vi "imaging gate sweep.vi"() -> ()   [LabVIEW 2021]
uses:
  <userlib>/Nanonis Prog Interface V5/Nanonis Prog Interface.lvlib
panel:
  in  "Home\nafter?":bool
  in  "?":bool
  in  "milliseconds to wait":u32
  in  "Direction: \nUp\n\n\nDown":bool=TRUE
  in  "Serie name":string caption="Basename (empty= no change)"
  in  "Gate increment (V)":dbl
  in  "End gate (V)":dbl
  in  "Start gate (V)":dbl
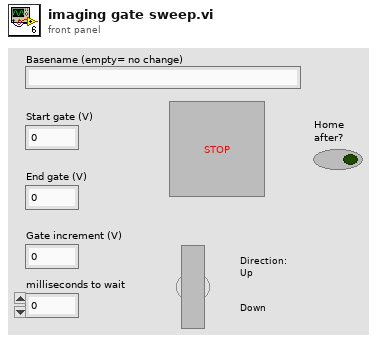
[diagram p1: front panel]
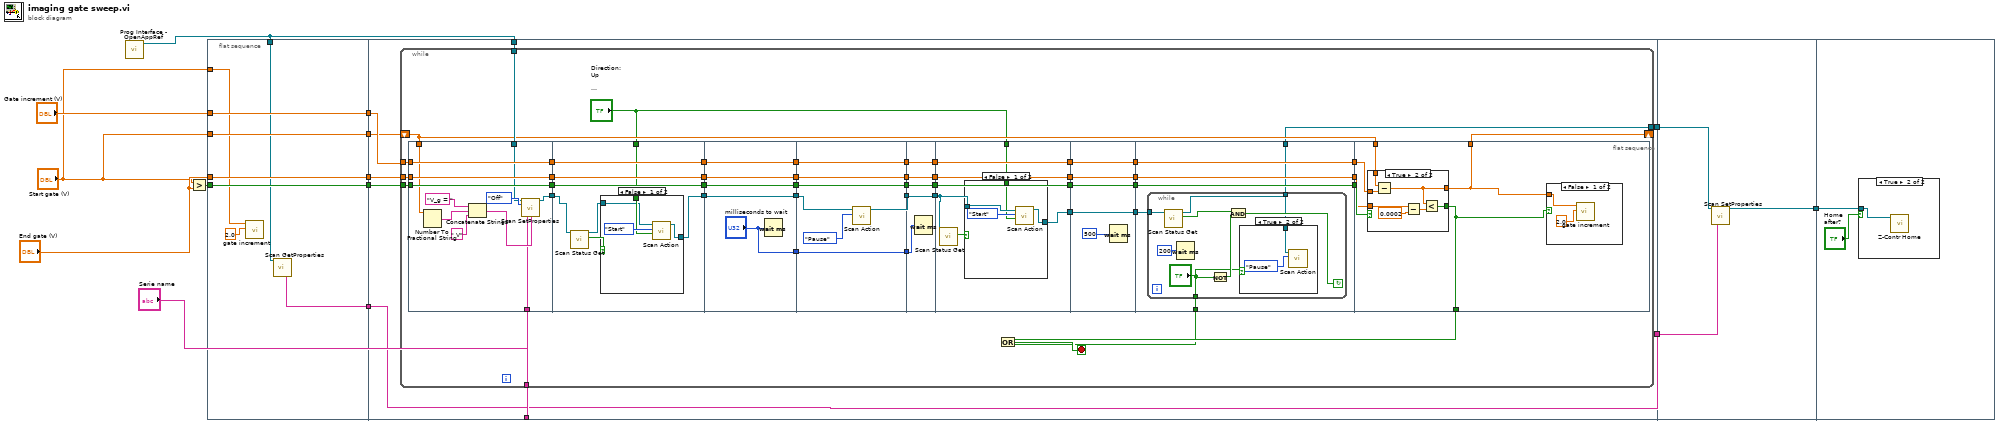
[diagram p0: block diagram]
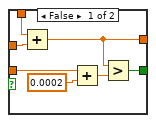
[diagram p6: hidden frame]
diagram:
  n1 = call <userlib>:"Prog Interface - OpenAppRef.vi"() -> ("Application reference"=w3:refnum<vi>)  [unwired: 6 in, 1 out]
  n2 = Greater?(x="Start gate (V)", y="End gate (V)") -> (0:w14:bool)
  n3 = flat-sequence {
    tunnel: "End gate (V)" -> [w19]
    tunnel: "Start gate (V)" -> [w20]
    tunnel: "Gate increment (V)" -> [w21]
    tunnel: w14 -> [w22]
    tunnel: [w22] -> w11
    tunnel: [w21] -> w10
    tunnel: [w20] -> w9
    tunnel: [w19] -> w8
    tunnel: "Start gate (V)" -> [w17]
    tunnel: [w16] -> w5
    tunnel: w3 -> [w15]
    tunnel: w11 -> [w30]
    tunnel: w10 -> [w29]
    tunnel: w9 -> [w28]
    tunnel: w8 -> [w27]
    tunnel: w3 -> [w26]
    tunnel: "Serie name" -> [w25]
    tunnel: w5 -> [w24]
    tunnel: [w24] -> w4
    tunnel: [w23] -> w2
    tunnel: w4 -> [w174]
    tunnel: w2 -> [w173]
    tunnel: [w172] -> w1
    tunnel: w1 -> [w176]
    frame #0 {
      n4 = call "gate increment.vi"("Increment"=2.0, "Gate Voltage"=w17) -> ()  [unwired: 10 in]
      n5 = call <userlib>:"Scan GetProperties.vi"("Application ref in"=w15) -> ("Serie name"=w16:string)  [unwired: 8 in, 6 out]
    }
    frame #1 {
      n6 = while {
        tunnel: w30 -> [w75]
        tunnel: w29 -> [w74]
        shift-right: [w66] -> _
        shift-left: w28 -> [w67]
        tunnel: w27 -> [w73]
        tunnel: w26 -> [w69]
        tunnel: w25 -> [w68]
        tunnel: [w39] -> w23
        stop <- w64 stop-if-true
        n7 = flat-sequence {
          tunnel: w73 -> [w85]
          tunnel: w74 -> [w86]
          tunnel: w75 -> [w87]
          tunnel: [w87] -> w62
          tunnel: [w86] -> w60
          tunnel: [w85] -> w58
          tunnel: w67 -> [w81]
          tunnel: w69 -> [w78]
          tunnel: [w77] -> w56
          tunnel: w68 -> [w76]
          tunnel: w62 -> [w95]
          tunnel: [w95] -> w61
          tunnel: w60 -> [w94]
          tunnel: [w94] -> w59
          tunnel: w58 -> [w93]
          tunnel: [w93] -> w57
          tunnel: w56 -> [w89]
          tunnel: [w90] -> w55
          tunnel: "Direction: \nUp\n\n\nDown" -> [w91]
          tunnel: w61 -> [w105]
          tunnel: [w105] -> w53
          tunnel: w59 -> [w104]
          tunnel: [w104] -> w52
          tunnel: w57 -> [w103]
          tunnel: [w103] -> w51
          tunnel: w55 -> [w102]
          tunnel: [w102] -> w50
          tunnel: ["milliseconds to wait"] -> w40
          tunnel: w53 -> [w112]
          tunnel: [w112] -> w49
          tunnel: w52 -> [w111]
          tunnel: [w111] -> w47
          tunnel: w51 -> [w110]
          tunnel: [w110] -> w45
          tunnel: w50 -> [w108]
          tunnel: [w107] -> w43
          tunnel: [w106] -> w41
          tunnel: w40 -> [w106]
          tunnel: w49 -> [w117]
          tunnel: [w117] -> w48
          tunnel: w47 -> [w116]
          tunnel: [w116] -> w46
          tunnel: w45 -> [w115]
          tunnel: [w115] -> w44
          tunnel: w43 -> [w114]
          tunnel: [w114] -> w42
          tunnel: w41 -> [w113]
          tunnel: w48 -> [w124]
          tunnel: [w124] -> w38
          tunnel: w46 -> [w123]
          tunnel: [w123] -> w36
          tunnel: w44 -> [w122]
          tunnel: [w122] -> w34
          tunnel: w42 -> [w119]
          tunnel: [w121] -> w32
          tunnel: "Direction: \nUp\n\n\nDown" -> [w118]
          tunnel: w38 -> [w134]
          tunnel: [w134] -> w37
          tunnel: w36 -> [w133]
          tunnel: [w133] -> w35
          tunnel: w34 -> [w132]
          tunnel: [w132] -> w33
          tunnel: w32 -> [w131]
          tunnel: [w131] -> w31
          tunnel: w37 -> [w140]
          tunnel: [w140] -> w72
          tunnel: w35 -> [w139]
          tunnel: [w139] -> w71
          tunnel: w33 -> [w138]
          tunnel: [w138] -> w70
          tunnel: w31 -> [w137]
          tunnel: [w136] -> w63
          tunnel: [w135] -> w39
          tunnel: w70 -> [w153]
          tunnel: w71 -> [w154]
          tunnel: w72 -> [w155]
          tunnel: [w152] -> w65
          tunnel: w67 -> [w151]
          tunnel: [w150] -> w66
          frame #0 {
            n8 = Number To Fractional String(number=w81) -> (F-format string=w84:string)  [unwired: 3 in]
            n9 = Concatenate Strings("V_g = " ("string"), w84, " V" ("string")) -> (w80:string)
            n10 = call <userlib>:"Scan SetProperties.vi"("Application ref in"=w78, "Continuous scan"=enum16{"No change", "On", "Off"}."Off", "Serie name"=w76, "Comment"=w80) -> ("Application ref out"=w77:refnum<vi>)  [unwired: 10 in, 1 out]
          }
          frame #1 {
            n11 = call <userlib>:"Scan Status Get.vi"("Application ref in"=w89) -> ("Scanning?"=w92:bool, "Application ref out"=w88:refnum<vi>)  [unwired: 7 in, 1 out]
            n12 = case shown="False" w92 {
              tunnel: [w98 w100] -> w90
              tunnel: w91 -> [w97 _]
              tunnel: w88 -> [w96 w100]
              frame False {
                n13 = call <userlib>:"Scan Action.vi"("Direction: up/down (T=up)"=w97, "Scan action (Start)"=enum16{"Start", "Stop", "Pause", "Resume"}."Start", "Application ref in"=w96) -> ("Application ref out"=w98:refnum<vi>)  [unwired: 6 in, 1 out]
              }
              frame True {
              }
            }
          }
          frame #2 {
            n14 = Wait (ms)(milliseconds to wait="milliseconds to wait") -> ()  [unwired: 1 out]
          }
          frame #3 {
            n15 = call <userlib>:"Scan Action.vi"("Scan action (Start)"=enum16{"Start", "Stop", "Pause", "Resume"}."Pause", "Application ref in"=w108) -> ("Application ref out"=w107:refnum<vi>)  [unwired: 7 in, 1 out]
          }
          frame #4 {
            n16 = Wait (ms)(milliseconds to wait=w113) -> ()  [unwired: 1 out]
          }
          frame #5 {
            n17 = call <userlib>:"Scan Status Get.vi"("Application ref in"=w119) -> ("Scanning?"=w120:bool)  [unwired: 7 in, 2 out]
            n18 = case shown="False" w120 {
              tunnel: w119 -> [w127 w129]
              tunnel: [w126 w129] -> w121
              tunnel: w118 -> [w125 _]
              frame False {
                n19 = call <userlib>:"Scan Action.vi"("Direction: up/down (T=up)"=w125, "Scan action (Start)"=enum16{"Start", "Stop", "Pause", "Resume"}."Start", "Application ref in"=w127) -> ("Application ref out"=w126:refnum<vi>)  [unwired: 6 in, 1 out]
              }
              frame True {
              }
            }
          }
          frame #6 {
            n20 = Wait (ms)(milliseconds to wait=u32 500) -> ()  [unwired: 1 out]
          }
          frame #7 {
            n21 = while {
              tunnel: w137 -> [w146]
              tunnel: ["?"] -> w136
              tunnel: [w141] -> w135
              stop <- w143 continue-if-true
              n22 = call <userlib>:"Scan Status Get.vi"("Application ref in"=w146) -> ("Scanning?"=w145:bool, "Application ref out"=w141:refnum<vi>)  [unwired: 7 in, 1 out]
              n23 = Wait (ms)(milliseconds to wait=u32 200) -> ()  [unwired: 1 out]
              n24 = Not(x="?") -> (.not. x?=w144:bool)
              n25 = And(x=w145, y=w144) -> (x .and. y?=w143:bool)
              n26 = case shown="True" "?" {
                tunnel: w141 -> [_ w148]
                frame False {
                }
                frame True {
                  n27 = call <userlib>:"Scan Action.vi"("Scan action (Start)"=enum16{"Start", "Stop", "Pause", "Resume"}."Pause", "Application ref in"=w148) -> ()  [unwired: 7 in, 2 out]
                }
              }
            }
          }
          frame #8 {
            n28 = case shown="True" w155 {
              tunnel: w154 -> [w164 w171]
              tunnel: [w159 w169] -> w150
              tunnel: w153 -> [w163 w168]
              tunnel: [w161 w170] -> w152
              tunnel: w151 -> [w158 w165]
              frame False {
                n29 = Add(x=w158, y=w164) -> (x+y=w159:dbl)
                n30 = Add(x=w163, y=0.0002) -> (x+y=w160:dbl)
                n31 = Greater?(x=w159, y=w160) -> (0:w161:bool)
              }
              frame True {
                n32 = Subtract(x=w165, y=w171) -> (x-y=w169:dbl)
                n33 = Subtract(x=w168, y=0.0002) -> (x-y=w166:dbl)
                n34 = Less?(x=w169, y=w166) -> (x < y?=w170:bool)
              }
            }
            n35 = case shown="False" w152 {
              tunnel: w150 -> [w157 _]
              frame False {
                n36 = call "gate increment.vi"("Increment"=2.0, "Gate Voltage"=w157) -> ()  [unwired: 10 in]
              }
              frame True {
              }
            }
          }
        }
        n37 = Or(x=w65, y=w63) -> (x .or. y?=w64:bool)
      }
    }
    frame #2 {
      n38 = call <userlib>:"Scan SetProperties.vi"("Application ref in"=w173, "Serie name"=w174) -> ("Application ref out"=w172:refnum<vi>)  [unwired: 12 in, 1 out]
    }
    frame #3 {
      n39 = case shown="True" "Home\nafter?" {
        tunnel: w176 -> [_ w177]
        frame False {
        }
        frame True {
          n40 = call <userlib>:"Z-Contr Home.vi"("Application ref in"=w177) -> ()  [unwired: 9 in, 2 out]
        }
      }
    }
  }
